vi "Encode32bitWrite.vi"(10 "Numeric":i32=1234567890) -> (2 "PololuString":string)   [LabVIEW 2018]
panel:
  out "MSBsByte":bool[](array[boolean])
  out "individualBytes":bool[][](array[boolean])
  out "hexBytes":u32[](array[numeric]) format="%02x"
  out "32bits":bool[](array[boolean])
  # "https://www.pololu.com/docs/0J71/9"
  # "LSB"
  # "MSB"
  # "data1"
  # "data2"
  # "data3"
  # "data4"
  # "LSB"
  # "MSB"
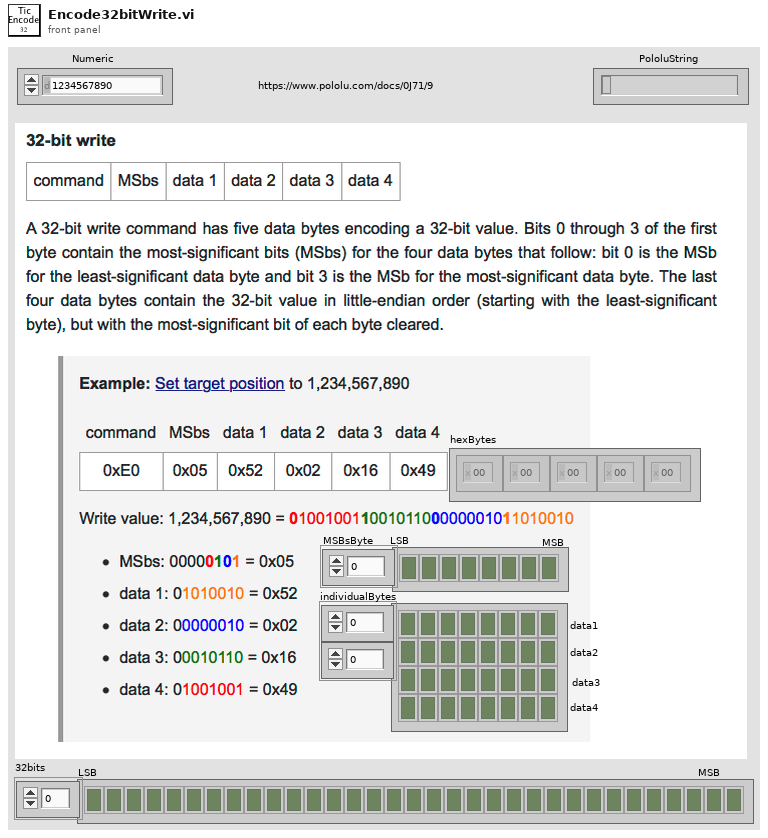
[diagram p1: front panel]
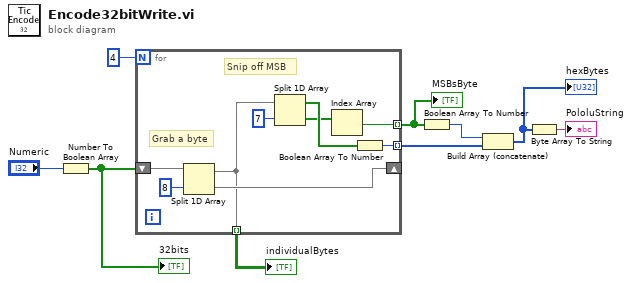
[diagram p0: block diagram]
diagram:
  n1 = Number To Boolean Array(number="Numeric") -> (Boolean array=w8:bool[])
  "32bits" <- w8
  n2 = for {
    N: 4 -> [_]
    shift-right: [w16] -> _
    shift-left: w8 -> [w13]
    tunnel: [w14] -> w1 mode=indexing
    tunnel: [w15] -> w5 mode=indexing
    tunnel: [w10] -> w2 mode=indexing
    # "Snip off MSB"
    # "Grab a byte"
    n3 = Split 1D Array(array=w13, index=8 ("length")) -> (first subarray=w10:bool[], second subarray=w16:bool[])
    n4 = Split 1D Array(array=w10, index=7 ("length")) -> (first subarray=w12:bool[], second subarray=w11:bool[])
    n5 = Index Array(array=w11) -> (element=w14:bool)  [unwired: 1 in]
    n6 = Boolean Array To Number(Boolean array=w12) -> (number=w15:u32)
  }
  "individualBytes" <- w2
  "MSBsByte" <- w1
  n7 = Boolean Array To Number(Boolean array=w1) -> (number=w6:u32)
  n8 = Build Array (concatenate)(w6, w5) -> (w4:u32[])
  "hexBytes" <- w4
  n9 = Byte Array To String(unsigned byte array=w4) -> (string=→"PololuString":string)
